vi "determineConPanePattern.vi"() -> ()   [LabVIEW 2017, in "vi_tools.lvlib"]
doc: "Select a Connector Pane pattern in the ring to find out the pattern number."
uses:
  vi_tools.lvlib
panel:
  out "Pattern Value":u32
  in  "Connector Panes":u16(ring)=3
  # "Select a Connector Pane pattern in the ring \nto find out the pattern number."
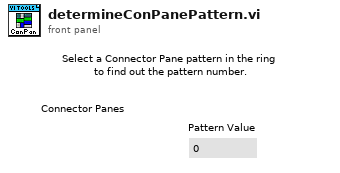
[diagram p1: front panel]
types:
  T1 = enum32{"Invalid", "Standard", "Closed", "Hidden", "Minimized", "Maximized"}
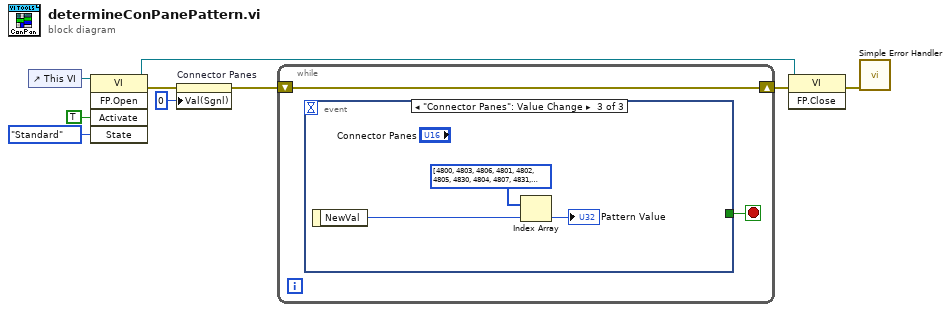
[diagram p0: block diagram]
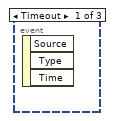
[diagram p2: hidden frame]
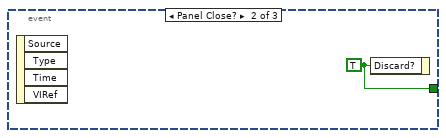
[diagram p3: hidden frame]
diagram:
  n1 = control-ref of="This VI"() -> (w5:refnum<vi>)
  n2 = invoke class="VI" method="FP.Open"(reference=w5, "Activate"=TRUE ("Activate?"), "State"=T1."Standard") -> (reference out=w6:refnum<vi>, error out=w3:errorcluster)  [unwired: 2 in, 3 out]
  n3 = property on="Connector Panes" class="Ring (strict)"(error in=w3, "Val(Sgnl)"=u16 0 ("Value (Signaling)")) -> (error out=w2:errorcluster)  [unwired: 1 in, 1 out]
  n4 = while {
    shift-right: [w10] -> w7
    shift-left: w2 -> [w10]
    stop <- w11 stop-if-true
    n5 = event shown="[2] \"Connector Panes\": Value Change" {
      selector: _ -> [_ _ _]
      dyn-events: _ -> [_ _ _]
      timeout: _ -> [_ _ _]
      tunnel: [_ w12 _] -> w11
      event Timeout {
        n6 = event-data() -> ()  [unwired: 1 in, 3 out]
      }
      event Panel Close? {
        w12 = TRUE ("Discard?")
        n7 = event-data() -> ()  [unwired: 1 in, 4 out]
        n8 = event-data("Discard?"=w12) -> ()  [unwired: 1 in, 1 out]
      }
      event "Connector Panes": Value Change {
        n9 = event-data() -> ("NewVal"=w13:u16)  [unwired: 1 in]
        n10 = Index Array(array=u32[] [4800, 4803, 4806, 4801, 4802, 4805, 4830, 4804, 4807, 4831, 4832, 4810, 4808, 4809, 4811, 4812, 4816, 4823, 4824, 4817, 4818, 4825, 4819, 4813, 4820, 4826, 4821, 4827, 4828, 4822, 4814, 4829, 4815, 4833, 4834, 4835], index=w13) -> (element=→"Pattern Value":u32)
      }
    }
  }
  n11 = invoke class="VI" method="FP.Close"(reference=w6, error in=w7) -> (error out=w4:errorcluster)  [unwired: 1 in, 2 out]
  n12 = call <vilib>:"Simple Error Handler.vi"("error in (no error)"=w4) -> ()  [unwired: 4 in, 5 out]
